vi "Arrange Work Terminals.vi"(9 "Work Types":T1[](array[typedef]), 10 "Work Terminals":refnum<vi>[](array[refnum]), 11 "VI":refnum<vi>) -> (0 "error out":errorcluster)   [LabVIEW 2020, in "FlexBlocks.lvlib"]
uses:
  FlexBlocks.lvlib
  Terminal Config.ctl
  Type Descriptor.ctl
  Terminal Direction.ctl
  Value Mode.ctl
  Special Terminal.ctl
  Terminal Mode.ctl
  <vilib>/Utility/traverseref.llb/TRef TravTarget.ctl
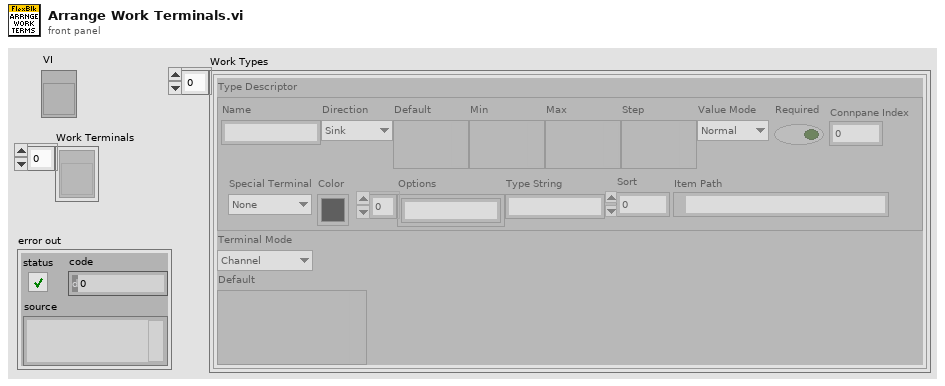
[diagram p1: front panel]
types:
  T1 = typedef "FlexBlocks.lvlib/Terminal Config.ctl" = cluster{"Type Descriptor":T2, "Terminal Mode":T6, "Default":variant}
  T2 = typedef "FlexBlocks.lvlib/Type Descriptor.ctl" = cluster{"Name":string, "Direction":T3, "Default":variant, "Min":variant, "Max":variant, "Step":variant, "Value Mode":T4, "Required":bool, "Connpane Index":i32, "Special Terminal":T5, "Color":u32, "Options":string[], "Type String":string, "Sort":i32, "Item Path":path}
  T3 = typedef "FlexBlocks.lvlib/Terminal Direction.ctl" = enum16{"Sink", "Source"}
  T4 = typedef "FlexBlocks.lvlib/Value Mode.ctl" = enum16{"Normal", "Range", "Select"}
  T5 = typedef "FlexBlocks.lvlib/Special Terminal.ctl" = enum16{"None", "Action", "Init", "Tag", "State in", "State out", "Error"}
  T6 = typedef "FlexBlocks.lvlib/Terminal Mode.ctl" = enum16{"Channel", "Config", "Value", "Control Ref"}
  T7 = typedef "TRef TravTarget.ctl" = enum16{"FP", "BD", "Other"}
  T8 = typedef "LVPositionTypeDef.ctl" = cluster{"Left":i32, "Top":i32}
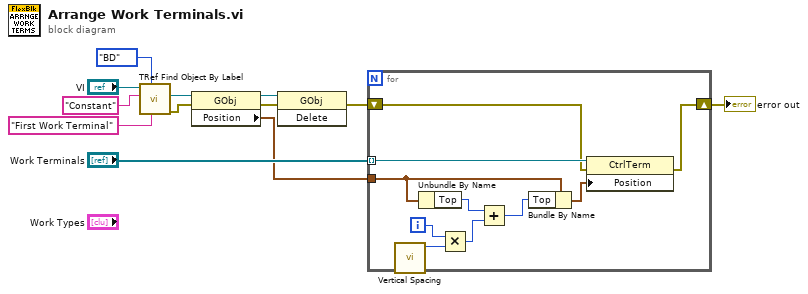
[diagram p0: block diagram]
diagram:
  n1 = call <vilib>:"TRef Find Object By Label.vi"("Label"="First Work Terminal", "Traverse Target"=TRef_TravTarget."BD", "Class Name"="Constant", "VI Ref"="VI") -> ("error out"=w7:errorcluster, "Found Obj Ref"=w9:refnum<vi>)  [unwired: 4 in, 2 out]
  n2 = property class="GObj"(reference=w9, error in=w7) -> (reference out=w8:refnum<vi>, error out=w6:errorcluster, "Position"=w2:T8)
  n3 = invoke class="GObj" method="Delete"(reference=w8, error in=w6) -> (error out=w4:errorcluster)  [unwired: 1 in, 2 out]
  n4 = for {
    tunnel: "Work Terminals" -> [w22] mode=indexing
    tunnel: w2 -> [w21]
    shift-right: [w14] -> w1
    shift-left: w4 -> [w15]
    i -> [w20]
    n5 = call "Vertical Spacing.vi"() -> ("Spacing"=w13:i32)  [unwired: 11 in]
    n6 = Unbundle By Name(w21) -> ("Top"=w19:i32)
    n7 = Multiply(x=w20, y=w13) -> (x*y=w18:i32)
    n8 = Add(x=w19, y=w18) -> (x+y=w17:i32)
    n9 = Bundle By Name(cluster=w21, "Top"=w17) -> (w16:T8)
    n10 = property class="CtrlTerm"(reference=w22, error in=w15, "Position"=w16) -> (error out=w14:errorcluster)  [unwired: 1 out]
  }
  "error out" <- w1
